vi "Get Objects.vi"(8 "error in (no error)":errorcluster, 11 "session in":refnum<k35>) -> (0 "error out":errorcluster, 3 "childs":string[](array[string]))   [LabVIEW 2019]
panel:
  out "session out":refnum<k35>
  out "Success":bool
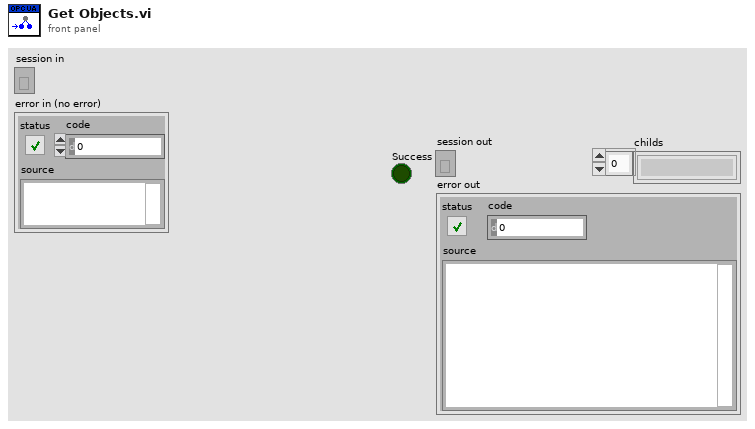
[diagram p1: front panel]
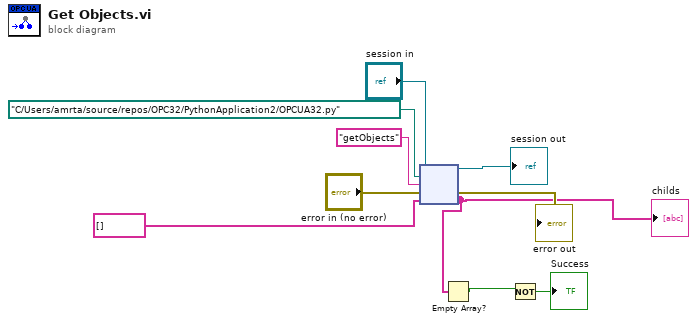
[diagram p0: block diagram]
diagram:
  n1 = node("session in", path "C:/Users/amrta/source/repos/OPC32/PythonApplication2/OPCUA32.py" ("module path"), "getObjects" ("function name"), "error in (no error)", string[] []) -> (→"session out":refnum<k35>, →"error out":errorcluster, w1:string[])  [unwired: 2 out]
  "childs" <- w1
  n2 = Empty Array?(array=w1) -> (empty?=w2:bool)
  n3 = Not(x=w2) -> (.not. x?=→"Success":bool)
